vi "BooleanToOnOff(array).vi"(11 "Enabled (array)":bool[](array[boolean])) -> (3 "Array":T1[](array[typedef]))   [LabVIEW 2011]
uses:
  OnOffTypeDef.ctl
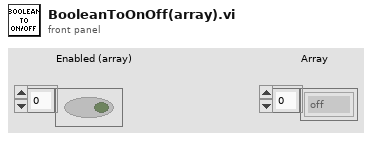
[diagram p1: front panel]
types:
  T1 = typedef "OnOffTypeDef.ctl" = enum16{"off", "on"}
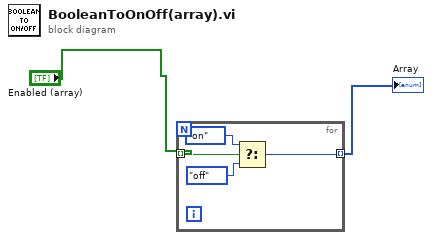
[diagram p0: block diagram]
diagram:
  n1 = for {
    tunnel: "Enabled (array)" -> [w6] mode=indexing
    tunnel: [w3] -> w2 mode=indexing
    n2 = Select(t=OnOffTypeDef."on" ("Channel 0"), s=w6, f=OnOffTypeDef."off" ("Channel 0")) -> (s? t:f=w3:T1)
  }
  "Array" <- w2
